vi "Mass_Qualitative_IV_Reader.vi"() -> ()   [LabVIEW 2016]
uses:
  <userlib>/LevyLab/LV to ITX/LVtoITX.lvclass
panel:
  in  "Points to chop off the bottom edge":i32
  in  "Points to chop off the top edge":i32
  out "current subfolder":path
  in  "Path to PNG Folder":path
  in  "e^2/h ?":bool
  in  "X step":dbl
  in  "X start":dbl
  out "Differential Conductance":dbl[][](graph)=[[172.002], [172.014], [172.02], [172.032], [172.05], [172.038], [171.99], [171.984], [172.008], [172.02], [172.038], [172.032], [172.008], [171.99], [171.984], [171.99], [172.008], [172.02], [172.032], [171.996], [172.002], [172.014], [172.032], [172.056], [172.056], [172.038], [172.008], [171.996], [172.014], [172.026], [172.032], [172.044], [172.008], [171.996], [171.99], [172.014], [172.032], [172.038], [172.032], [171.99], [171.984], [171.996], [172.014], [172.032], [172.026], [172.002], [171.99], [171.996], [172.02], [172.038], [172.05], [172.032], [172.002], [172.008], [172.014], [172.032], [172.044], [172.056], [172.044], [172.002], [171.996], [172.002], [172.026], [172.038], [172.044], [172.05], [172.02], [172.002], [171.99], [172.002], [172.008], [172.026], [172.02], [171.978], [171.978], [171.984], [171.99], [171.99], [172.002], [171.978], [171.96], [171.972], [171.984], [171.99], [171.996], [171.996], [171.978], [171.954], [171.948], [171.972], [171.99], [172.008], [172.032], [172.014], [171.996], [172.008], [172.014], [172.014], [172.008], [171.99], [171.972], [171.972], [171.99], [172.008], [172.032], [172.02], [171.996], [171.984], [171.996], [172.014], [172.02], [172.002], [171.972], [171.978], [171.99], [172.008], [172.026], [172.026], [171.99], [171.978], [171.99], [171.996], [172.002], [172.002], [172.002]]
  in  "Portion of data":cluster{dbl, dbl}(slide)={0.75, 0.25} scale=0.0..1.0
  out "hmmmm":cluster{dbl[], dbl[]}(graph)
  out "Iterations of loop":i32
  out "directory":bool
  out "dI/dV":cluster{dbl[], dbl[]}[](graph)
  out "A vs B":cluster{dbl[], dbl[]}[](graph)
  in  "Diff bin size":dbl
  out "Comments":string
  in  "Diff bin size":dbl=2.0
  out "N__":cluster{"N1":dbl, "N2":dbl, "N3":dbl, "N4":dbl}={"N1"=0.0624995231628418, "N2"=0.0624995231628418, "N3"=0.0624995231628418, "N4"=0.0624995231628418} {"N4" format="%#_6p"; "N3" format="%#_6p"; "N2" format="%#_6p"; "N1" format="%#_6p"}
  out "IV":dbl[][](graph)=[[172.002], [172.014], [172.02], [172.032], [172.05], [172.038], [171.99], [171.984], [172.008], [172.02], [172.038], [172.032], [172.008], [171.99], [171.984], [171.99], [172.008], [172.02], [172.032], [171.996], [172.002], [172.014], [172.032], [172.056], [172.056], [172.038], [172.008], [171.996], [172.014], [172.026], [172.032], [172.044], [172.008], [171.996], [171.99], [172.014], [172.032], [172.038], [172.032], [171.99], [171.984], [171.996], [172.014], [172.032], [172.026], [172.002], [171.99], [171.996], [172.02], [172.038], [172.05], [172.032], [172.002], [172.008], [172.014], [172.032], [172.044], [172.056], [172.044], [172.002], [171.996], [172.002], [172.026], [172.038], [172.044], [172.05], [172.02], [172.002], [171.99], [172.002], [172.008], [172.026], [172.02], [171.978], [171.978], [171.984], [171.99], [171.99], [172.002], [171.978], [171.96], [171.972], [171.984], [171.99], [171.996], [171.996], [171.978], [171.954], [171.948], [171.972], [171.99], [172.008], [172.032], [172.014], [171.996], [172.008], [172.014], [172.014], [172.008], [171.99], [171.972], [171.972], [171.99], [172.008], [172.032], [172.02], [171.996], [171.984], [171.996], [172.014], [172.02], [172.002], [171.972], [171.978], [171.99], [172.008], [172.026], [172.026], [171.99], [171.978], [171.99], [171.996], [172.002], [172.002], [172.002]]
  in  "index":T1={"A"=5, "B"=3, "C"=2, "D"=0, "E"=3, "N1"=0, "N2"=0, "N3"=0, "N4"=0}
  in  "SuperFolder":path=path "B:/SketchSET/SA03008H.20180718/08-BG_Sweep_-5to5_0.1_@0.1Hz"
  # "YES"
  # "NO"
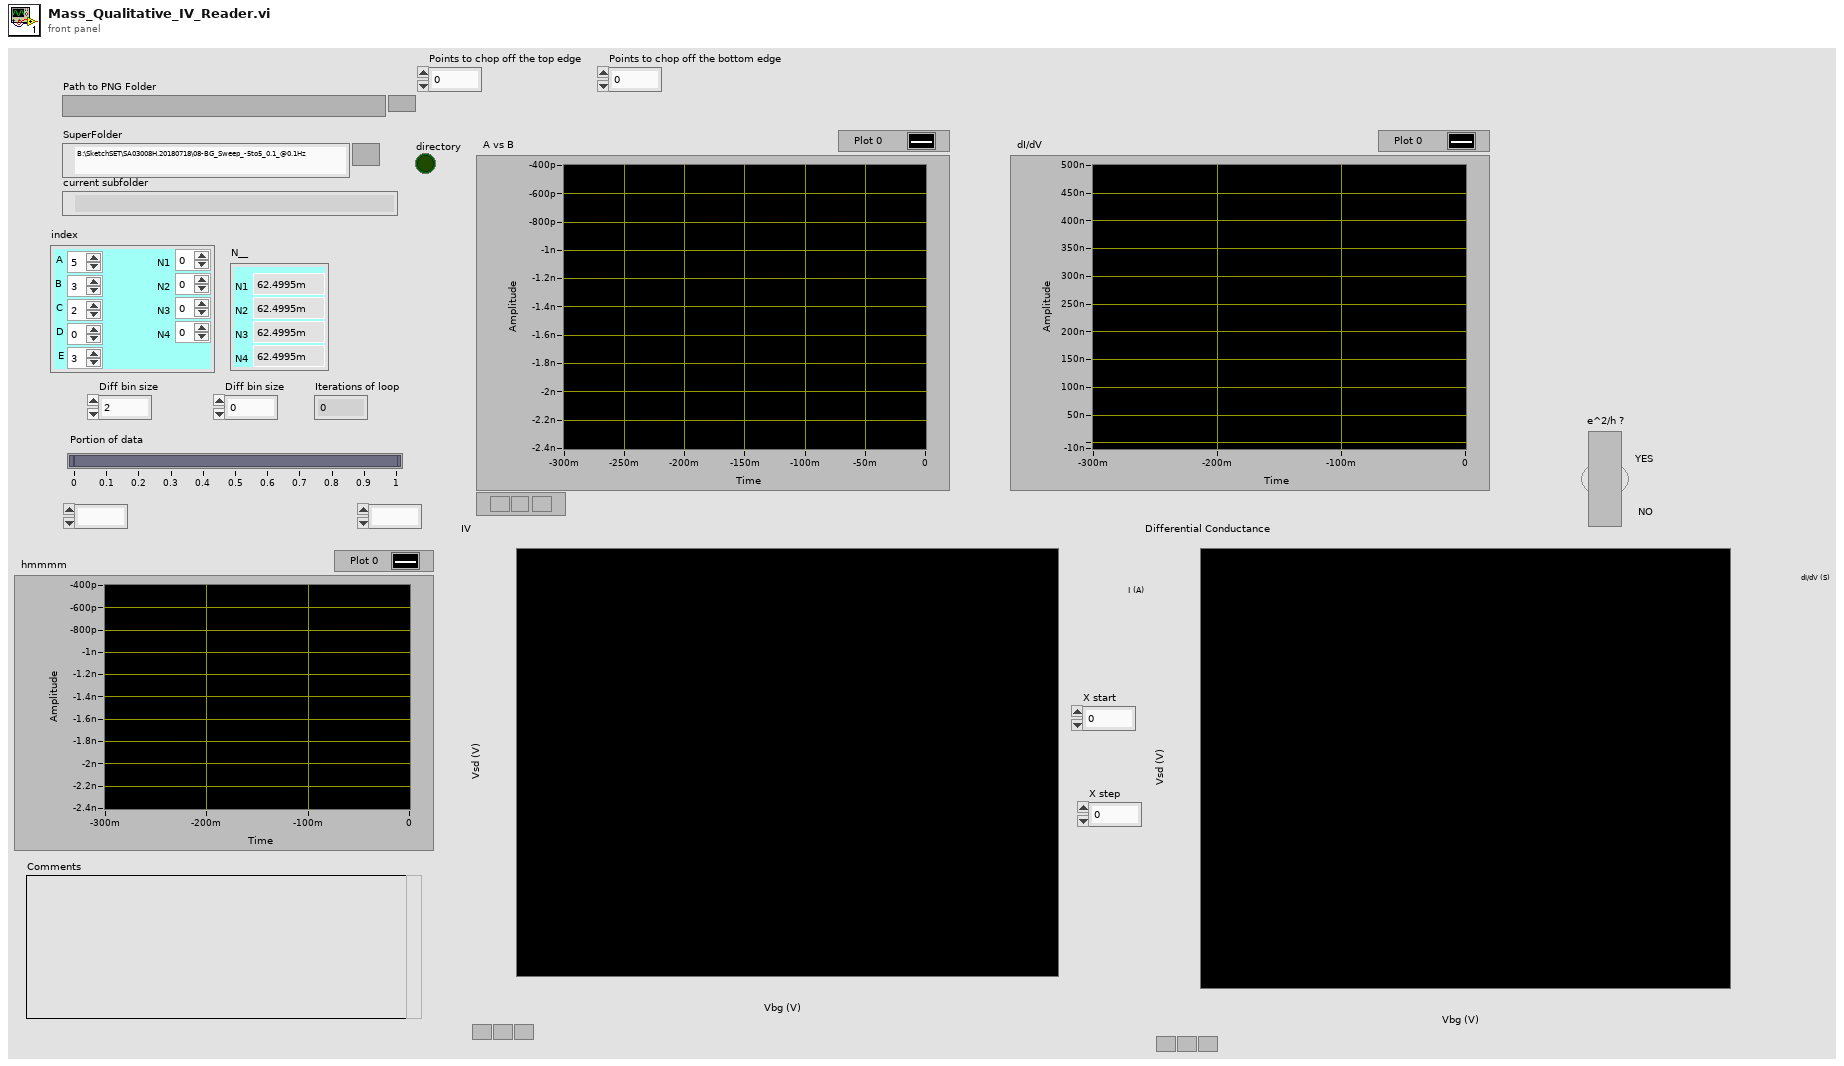
[diagram p1: front panel]
types:
  T1 = cluster{"A":i32, "B":i32, "C":i32, "D":i32, "E":i32, "N1":i32, "N2":i32, "N3":i32, "N4":i32}
  T2 = cluster{"Decimated Array":dbl[], "Decimated Array":dbl[]}[]
  T3 = cluster{"Decimated Array":dbl[], "Decimated Array":dbl[]}
  T4 = typedef "imagedata.ctl" = cluster{"image type":i32, "image depth":i32, "image":u8[], "mask":u8[], "colors":u32[], "Rectangle":cluster{"left":i16, "top":i16, "right":i16, "bottom":i16}}
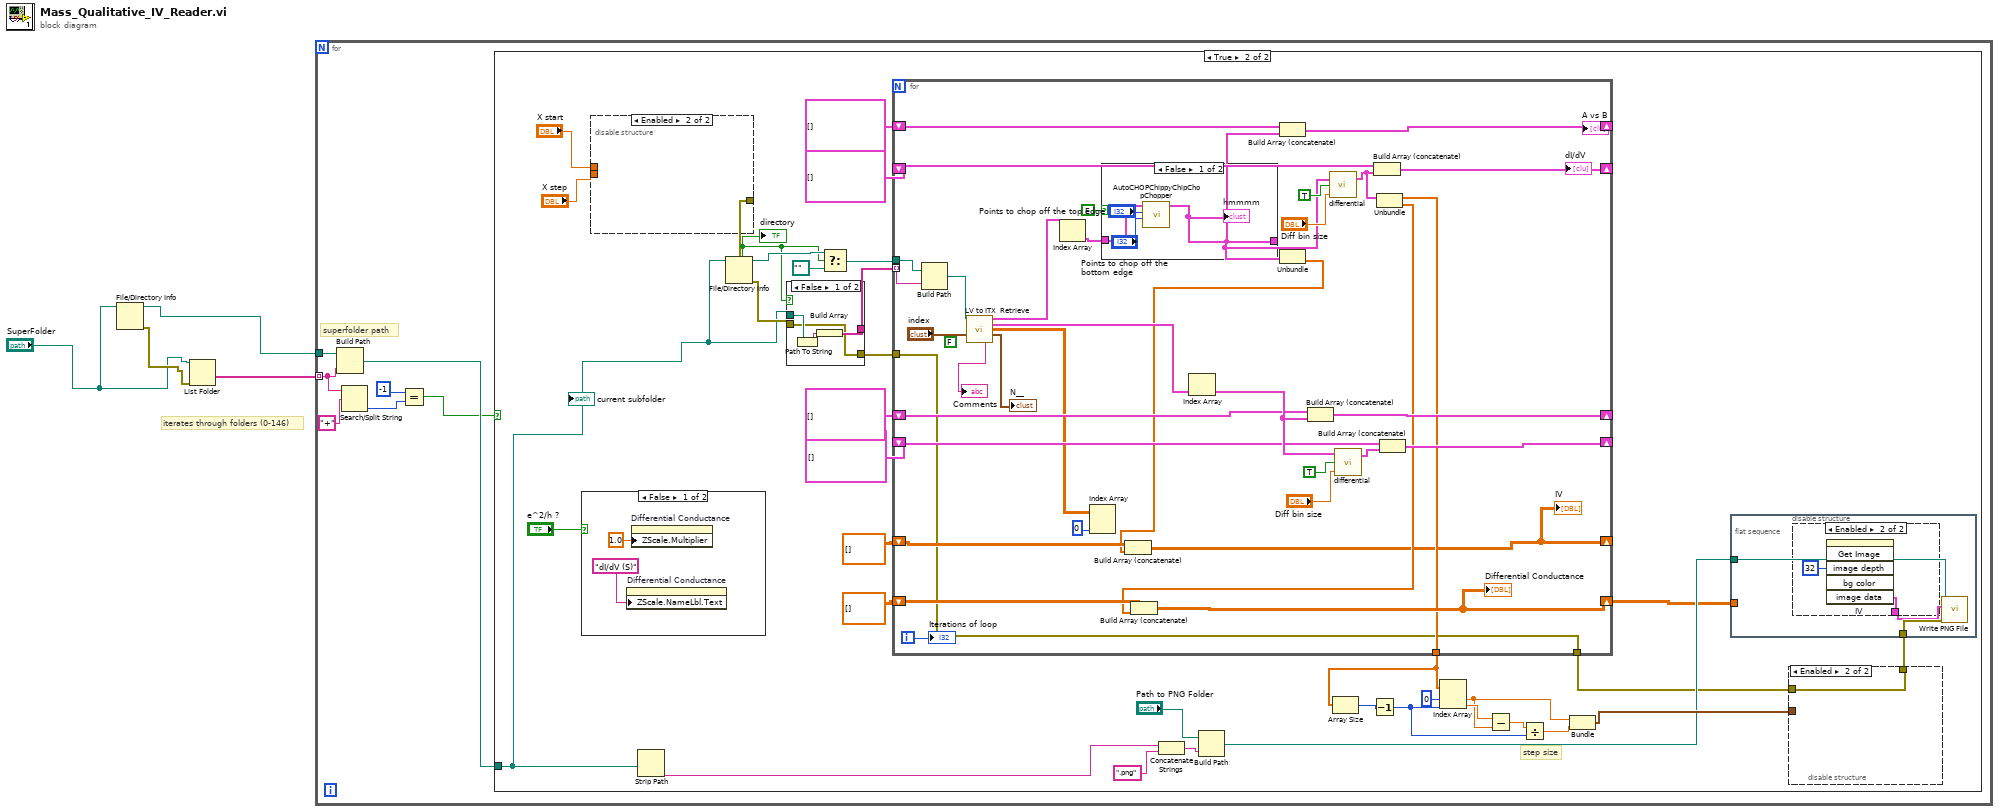
[diagram p0: block diagram]
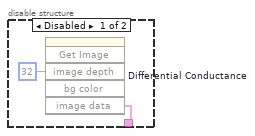
[diagram p3: hidden frame]
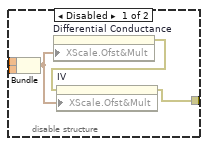
[diagram p4: hidden frame]
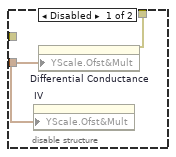
[diagram p5: hidden frame]
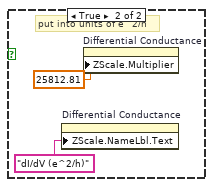
[diagram p6: hidden frame]
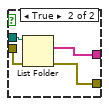
[diagram p7: hidden frame]
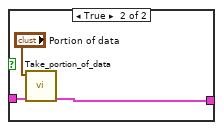
[diagram p8: hidden frame]
diagram:
  # "iterates through folders (0-146)"
  n1 = File/Directory Info(path="SuperFolder") -> (path out=w1:path, error out=w4:errorcluster)  [unwired: 1 in, 5 out]
  n2 = List Folder(path="SuperFolder", error in=w4) -> (folder names=w2:string[])  [unwired: 2 in, 3 out]
  n3 = for {
    tunnel: w2 -> [w10] mode=indexing
    tunnel: w1 -> [w11]
    # "superfolder path"
    n4 = Build Path(base path=w11, name or relative path=w10) -> (appended path=w6:path)
    n5 = Search/Split String(string=w10, search string/char (-)="+") -> (offset of match=w8:i32)  [unwired: 1 in, 2 out]
    n6 = Equal?(x=-1, y=w8) -> (x = y?=w5:bool)
    n7 = case shown="True" w5 {
      tunnel: w6 -> [_ w17]
      frame False {
      }
      frame True {
        # "step size"
        n8 = case shown="False" "e^2/h ?" {
          frame False {
            n9 = property on="Differential Conductance" class="IntGraph (strict)"("ZScale.NameLbl.Text"="dI/dV (S)" ("Z Scale.Unit Label.Text")) -> ()  [unwired: 2 in, 2 out]
            n10 = property on="Differential Conductance" class="IntGraph (strict)"("ZScale.Multiplier"=1.0 ("Z Scale.Offset and Multiplier:Multiplier")) -> ()  [unwired: 2 in, 2 out]
          }
          frame True {
            # "put into units of e^2/h"
            n11 = property on="Differential Conductance" class="IntGraph (strict)"("ZScale.NameLbl.Text"="dI/dV (e^2/h)" ("Z Scale.Unit Label.Text")) -> ()  [unwired: 2 in, 2 out]
            n12 = property on="Differential Conductance" class="IntGraph (strict)"("ZScale.Multiplier"=25812.81 ("Z Scale.Offset and Multiplier:Multiplier")) -> ()  [unwired: 2 in, 2 out]
          }
        }
        n13 = disable-structure shown="Enabled" {
          disable-tunnel: "X start" -> [w60 _]
          disable-tunnel: "X step" -> [w59 _]
          disable-tunnel: [w56 _] -> w23
          frame Disabled {
            n14 = Bundle("X start"=w60, "X step"=w59) -> (w58:cluster{"X start":dbl, "X step":dbl})  [unwired: 1 in]
            n15 = property on="Differential Conductance" class="IntGraph (strict)"("XScale.Ofst&Mult"=w58) -> (error out=w57:errorcluster)  [unwired: 2 in, 1 out]
            n16 = property on="IV" class="IntGraph (strict)"(error in=w57, "XScale.Ofst&Mult"=w58) -> (error out=w56:errorcluster)  [unwired: 1 in, 1 out]
          }
          frame Enabled {
          }
        }
        n17 = Strip Path(path=w17) -> (name=w15:string)  [unwired: 1 out]
        n18 = File/Directory Info(path=w17, error in=w23) -> (path out=w41:path, directory=w40:bool, error out=w43:errorcluster)  [unwired: 4 out]
        "directory" <- w40
        n19 = case shown="False" w40 {
          tunnel: w17 -> [w71 w75]
          tunnel: w43 -> [w68 w74]
          tunnel: [w69 w73] -> w42
          tunnel: [w68 w72] -> w14
          frame False {
            n20 = Path To String(path=w71) -> (string=w70:string)
            n21 = Build Array(w70) -> (w69:string[])
          }
          frame True {
            n22 = List Folder(path=w75, error in=w74) -> (filenames=w73:string[], error out=w72:errorcluster)  [unwired: 2 in, 2 out]
          }
        }
        n23 = Select(t=w41, s=w40, f=path "") -> (s? t:f=w39:path)
        n24 = for {
          shift-right: [w91] -> w36
          shift-left: cluster{dbl[], dbl[]}[] [] -> [w107]
          shift-right: [w97] -> w35
          shift-left: T2 [] -> [w106]
          shift-right: [w96] -> _
          shift-left: T2 [] -> [w101]
          shift-right: [w98] -> _
          shift-left: cluster{dbl[], dbl[]}[] [] -> [w100]
          tunnel: w42 -> [w79] mode=indexing
          shift-right: [w76] -> _
          shift-left: dbl[][] [] -> [w93]
          tunnel: w39 -> [w92]
          shift-right: [w81] -> w12
          shift-left: dbl[][] [] -> [w85]
          tunnel: [w80] -> w33
          tunnel: w14 -> [w78]
          tunnel: [w78] -> w13
          i -> [w90]
          (unwired) FALSE ("stop")
          n25 = Build Path(base path=w92, name or relative path=w79) -> (appended path=w99:path)
          n26 = call <userlib>:"LV to ITX  Retrieve.vi"("File or Folder Path"=w99, "index"="index") -> ("A vs B"=w87:cluster{dbl[], dbl[]}[], "C vs D"=w89:cluster{dbl[], dbl[]}[], "E"=w95:dbl[][], "N"=→"N__":cluster{"N1":dbl, "N2":dbl, "N3":dbl, "N4":dbl}, "Comments"=→"Comments":string)  [unwired: 9 in]
          n27 = Index Array(array=w87) -> (element=w86:cluster{dbl[], dbl[]})  [unwired: 1 in]
          n28 = Index Array(array=w95, index (col)=0 ("index (row)")) -> ()  [unwired: 1 in, 1 out]
          n29 = case shown="False" FALSE {
            tunnel: [w113 w118] -> w88
            tunnel: w86 -> [w116 w117]
            frame False {
              n30 = call "AutoCHOPChippyChipChopChopper.vi"("Points to chop off the bottom edge"="Points to chop off the bottom edge", "Points to chop off the top edge"="Points to chop off the top edge", "Vsrc and Current In"=w116) -> ("Vsrc and Current Out"=w113:cluster{dbl[], dbl[]})  [unwired: 8 in]
              "hmmmm" <- w113
            }
            frame True {
              n31 = call <userlib>:"Take_portion_of_data.vi"("input IV"=w117, "Slide"="Portion of data") -> ("Output IV"=w118:cluster{dbl[], dbl[]})  [unwired: 5 in]
            }
          }
          n32 = Index Array(array=w89) -> (element=w104:cluster{dbl[], dbl[]})  [unwired: 1 in]
          n33 = Build Array (concatenate)(w107, w88) -> (w91:cluster{dbl[], dbl[]}[])
          n34 = Unbundle(w88) -> (w82:dbl[])  [unwired: 1 out]
          n35 = Build Array (concatenate)(w93, w82) -> (w76:dbl[][])
          "IV" <- w76
          n36 = Build Array (concatenate)(w100, w104) -> (w98:cluster{dbl[], dbl[]}[])
          n37 = call <userlib>:"differential.vi"("Numeric"="Diff bin size", "dy/dx vs x"=TRUE, "A vs B 2"=w88) -> ("A vs B 3"=w84:T3)  [unwired: 1 in]
          n38 = call <userlib>:"differential.vi"("Numeric"="Diff bin size", "dy/dx vs x"=TRUE, "A vs B 2"=w104) -> ("A vs B 3"=w105:T3)  [unwired: 1 in]
          n39 = Build Array (concatenate)(w106, w84) -> (w97:T2)
          n40 = Unbundle(w84) -> ("Decimated Array"=w80:dbl[], "Decimated Array"=w83:dbl[])
          n41 = Build Array (concatenate)(w85, w83) -> (w81:dbl[][])
          "Differential Conductance" <- w81
          n42 = Build Array (concatenate)(w101, w105) -> (w96:T2)
          "Iterations of loop" <- w90
        }
        "A vs B" <- w36
        "dI/dV" <- w35
        n43 = Concatenate Strings(w15, ".png" ("string")) -> (w20:string)
        n44 = Build Path(base path="Path to PNG Folder", name or relative path=w20) -> (appended path=w18:path)
        n45 = Array Size(array=w33) -> (size(s)=w30:i32)
        n46 = Decrement(x=w30) -> (x-1=w29:i32)
        n47 = Index Array(array=w33, index #1=0 ("index"), index #2=w29) -> (element #1=w28:dbl, element #2=w32:dbl)
        n48 = Subtract(x=w32, y=w28) -> (x-y=w31:dbl)
        n49 = Divide(x=w31, y=w29) -> (x/y=w27:dbl)
        n50 = Bundle(w28, w27) -> (w24:cluster{dbl, dbl})  [unwired: 1 in]
        n51 = flat-sequence {
          tunnel: w18 -> [w51]
          tunnel: w16 -> [w50]
          tunnel: w12 -> [_]
          frame #0 {
            n52 = disable-structure shown="Enabled" {
              disable-tunnel: [w53 w54] -> w49
              frame Disabled {
                n53 = invoke on="Differential Conductance" class="IntGraph (strict)" method="Get Image"("image depth"=32 ("Image Depth")) -> ("image data"=w53:T4)  [unwired: 5 in, 5 out]
              }
              frame Enabled {
                n54 = invoke on="IV" class="IntGraph (strict)" method="Get Image"("image depth"=32 ("Image Depth")) -> ("image data"=w54:T4)  [unwired: 5 in, 5 out]
              }
            }
            n55 = call <vilib>:"Write PNG File.vi"("error in (no error)"=w50, "image data"=w49, "path to PNG file"=w51) -> ()  [unwired: 7 in, 2 out]
          }
        }
        n56 = disable-structure shown="Enabled" {
          disable-tunnel: w24 -> [w62 _]
          disable-tunnel: [w61 w63] -> w16
          disable-tunnel: w13 -> [_ w63]
          frame Disabled {
            n57 = property on="IV" class="IntGraph (strict)"("YScale.Ofst&Mult"=w62) -> ()  [unwired: 2 in, 2 out]
            n58 = property on="Differential Conductance" class="IntGraph (strict)"("YScale.Ofst&Mult"=w62) -> (error out=w61:errorcluster)  [unwired: 2 in, 1 out]
          }
          frame Enabled {
          }
        }
        "current subfolder" <- w17
      }
    }
  }
